vi "daqio_Get_Specific_Device_Type.vi"(8 "error in (no error)":errorcluster, 11 "daq.io type in":T6={"daq.io ref"=refnum, "daq.io API Base"="http://dashboard.daq.io/api/v1", "Device Type Key"="", "Device Key"="", "Account ID"=""}) -> (0 "error out":errorcluster, 2 "Device Type":T1, 3 "daq.io type out":T6={"daq.io ref"=refnum, "daq.io API Base"="http://dashboard.daq.io/api/v1", "Device Type Key"="", "Device Key"="", "Account ID"=""})   [LabVIEW 2013, in "daqio minimal.lvlib"]
doc: "This VI returns the currently selected Device Type. If any changes were made to the device type, call this VI and refresh the FGV to have the most recent version locally."
uses:
  daqio minimal.lvlib
  _typedefs/daqio-Type.ctl
  <vilib>/httpClient/ClientHandle.ctl
  _typedefs/daqio-Device-Type-Info-return.ctl
  _typedefs/daqio-Channel-Type-POST-return.ctl
  _typedefs/daqio-Device.ctl
  _typedefs/daqio-Event-Type.ctl
  _typedefs/daqio-Tag-Type-POST-return.ctl
  <vilib>/Easy HTTP Client/Easy HTTP.lvlib
  <vilib>/httpClient/LabVIEWHTTPClient.lvlib
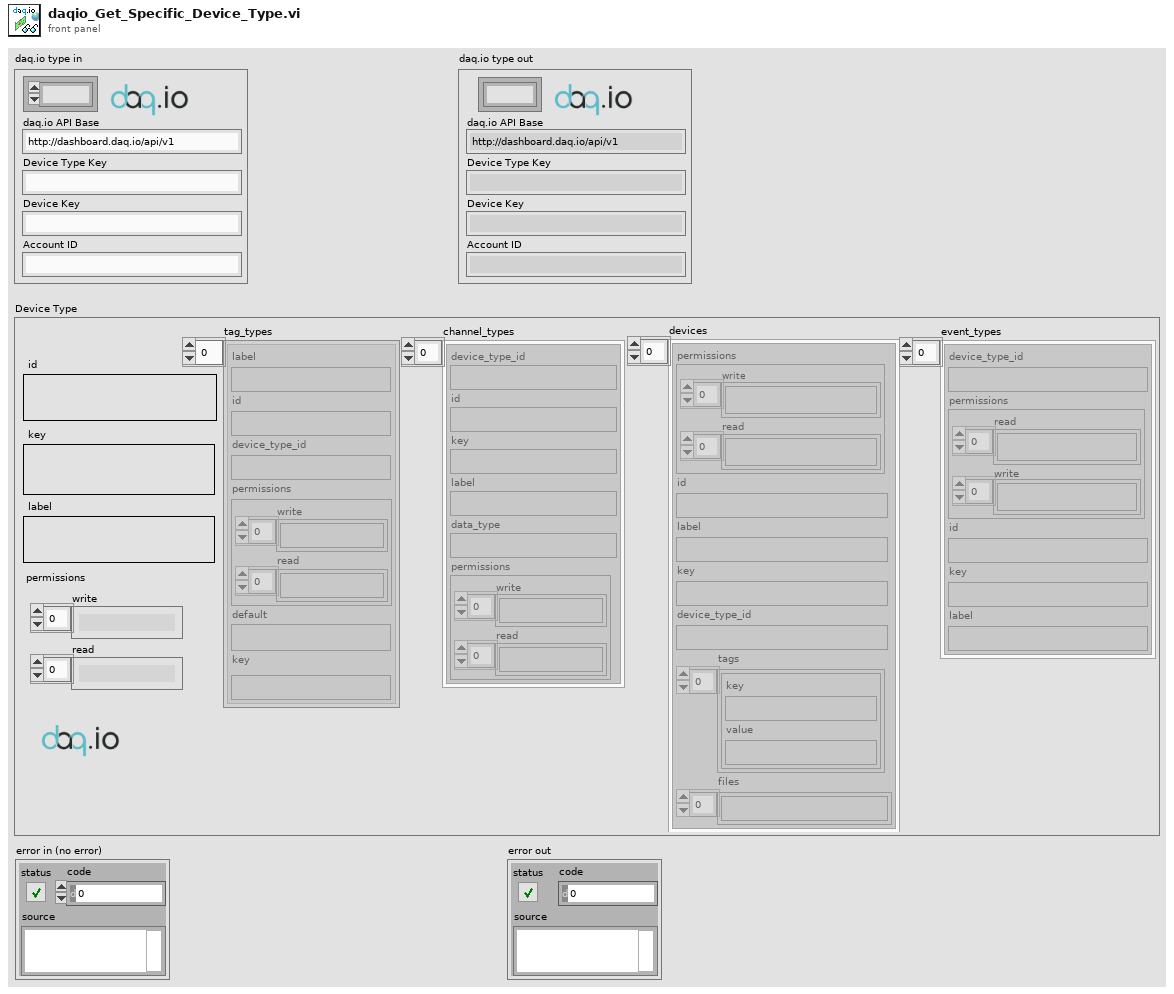
[diagram p1: front panel]
types:
  T1 = typedef "daqio minimal.lvlib/daqio-Device-Type-Info-return.ctl" = cluster{"channel_types":T2[], "devices":T3[], "label":string, "event_types":T4[], "key":string, "tag_types":T5[], "id":string, "permissions":cluster{"write":string[], "read":string[]}}
  T2 = typedef "daqio minimal.lvlib/daqio-Channel-Type-POST-return.ctl" = cluster{"device_type_id":string, "id":string, "key":string, "label":string, "data_type":string, "permissions":cluster{"write":string[], "read":string[]}}
  T3 = typedef "daqio minimal.lvlib/daqio-Device.ctl" = cluster{"permissions":cluster{"write":string[], "read":string[]}, "id":string, "label":string, "key":string, "device_type_id":string, "tags":cluster{"key":string, "value":string}[], "files":string[]}
  T4 = typedef "daqio minimal.lvlib/daqio-Event-Type.ctl" = cluster{"device_type_id":string, "permissions":cluster{"read":string[], "write":string[]}, "id":string, "key":string, "label":string}
  T5 = typedef "daqio minimal.lvlib/daqio-Tag-Type-POST-return.ctl" = cluster{"label":string, "id":string, "device_type_id":string, "permissions":cluster{"write":string[], "read":string[]}, "default":string, "key":string}
  T6 = typedef "daqio minimal.lvlib/daqio-Type.ctl" = cluster{"daq.io ref":T7, "daq.io API Base":string, "Device Type Key":string, "Device Key":string, "Account ID":string}
  T7 = typedef "LabVIEWHTTPClient.lvlib/ClientHandle.ctl" = refnum<k1>
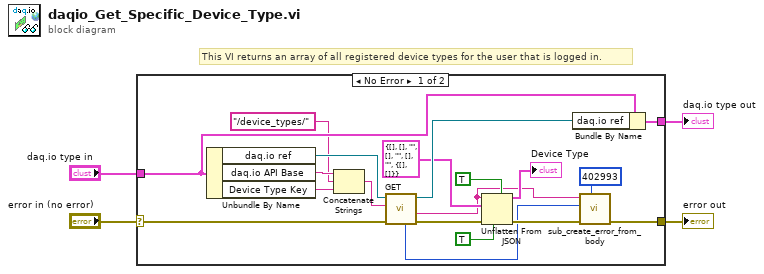
[diagram p0: block diagram]
diagram:
  # "This VI returns an array of all registered device types for the user that is logged in."
  n1 = case shown="No Error" "error in (no error)" {
    selector: "error in (no error)" -> [w19 w24]
    tunnel: "daq.io type in" -> [w23 w25]
    tunnel: [w22 w25] -> w3
    tunnel: [w8 w24] -> w2
    frame No Error {
      n2 = Unbundle By Name(w23) -> ("daq.io ref"=w21:T7, "daq.io API Base"=w17:string, "Device Type Key"=w11:string)
      n3 = Concatenate Strings(w17, "/device_types/", w11) -> (w15:string)
      n4 = call <vilib>:"GET.vi"("error in (no error)"=w19, "url"=w15, "client handle"=w21) -> ("error out"=w18:errorcluster, "body"=w5:string, "client handle out"=w20:T7, "HTTP Response Code"=w6:i32)  [unwired: 4 in, 1 out]
      n5 = Unflatten From JSON(enable LabVIEW extensions? (T)=TRUE, JSON string=w5, type and defaults=T1 {"channel_types"=[], "devices"=[], "label"="", "event_types"=[], "key"="", "tag_types"=[], "id"="", "permissions"={"write"=[], "read"=[]}} ("devices"), default null elements? (F)=TRUE, error in (no error)=w18) -> (value=→"Device Type":T1, error out=w9:errorcluster)  [unwired: 2 in]
      n6 = Bundle By Name(cluster=w23, "daq.io ref"=w20) -> (w22:T6)
      n7 = call "sub_create_error_from_body.vi"("error code"=402993, "error in (no error)"=w9, "http code"=w6, "body"=w5) -> ("error out"=w8:errorcluster)  [unwired: 7 in]
    }
    frame Error {
    }
  }
  "error out" <- w2
  "daq.io type out" <- w3
